vi "System State Global.vi"(7 "Notifier In":refnum<notifier>, 8 "Action":T2, 10 "State In":T1=enum."E-Stop") -> (0 "Notifier Out":refnum<notifier>, 2 "State Out":T1)   [LabVIEW 2015]
uses:
  System State Global Action.ctl
  System State.ctl
  Valve Button Mapping Global Action.ctl
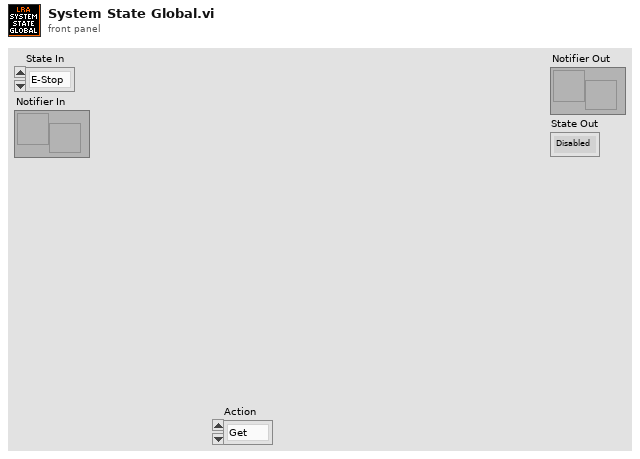
[diagram p1: front panel]
types:
  T1 = typedef "System State.ctl" = enum16{"Disabled", "E-Stop", "Standby", "Active"}
  T2 = typedef "System State Global Action.ctl" = enum16{"Get", "Set", "Initialize"}
  T3 = typedef "Valve Button Mapping Global Action.ctl" = enum16{"Get", "Set", "Init", "Reset All", "Reset to Standby"}
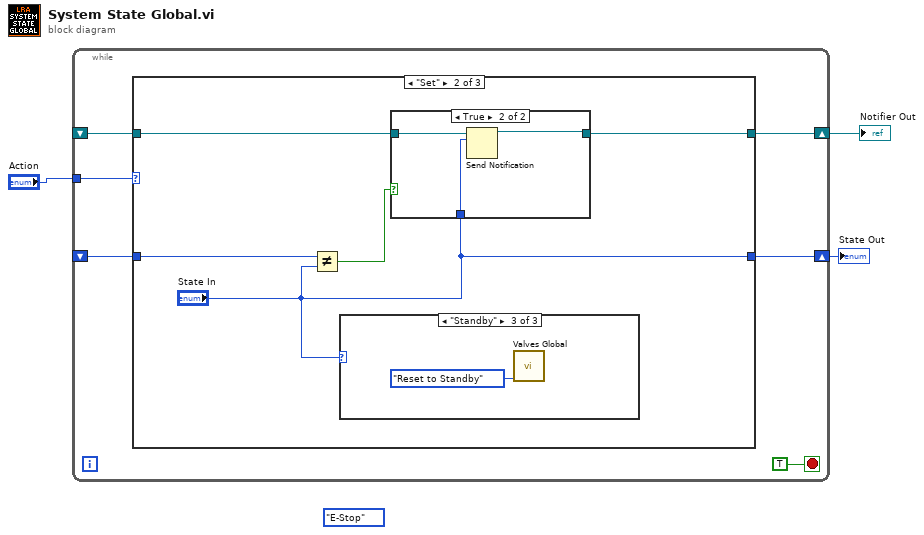
[diagram p0: block diagram]
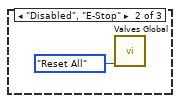
[diagram p4: hidden frame]
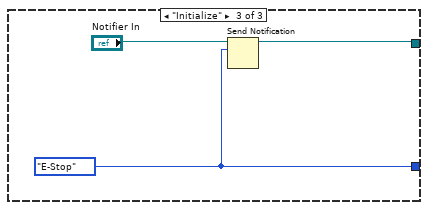
[diagram p6: hidden frame]
diagram:
  (unwired) System_State."E-Stop" ("notification")
  n1 = while {
    tunnel: "Action" -> [w8]
    shift-right: [w7] -> w1
    shift-left: _ -> [w6]
    shift-right: [w5] -> w2
    shift-left: _ -> [w4]
    stop <- TRUE stop-if-true
    n2 = case shown="\"Set\"" w8 {
      tunnel: [w11 "State In" w23] -> w7
      tunnel: w6 -> [w11 w16 _]
      tunnel: [w10 w13 w25] -> w5
      tunnel: w4 -> [w10 w14 _]
      frame "Get", Default {
      }
      frame "Set" {
        n3 = Not Equal?(x=w16, y="State In") -> (x != y?=w15:bool)
        n4 = case shown="\"Standby\"" "State In" {
          frame "Active", Default {
          }
          frame "Disabled", "E-Stop" {
            n5 = call "Valves Global.vi"("Action"=Valve_Button_Mapping_Global_Action."Reset All") -> ()  [unwired: 7 in, 4 out]
          }
          frame "Standby" {
            n6 = call "Valves Global.vi"("Action"=Valve_Button_Mapping_Global_Action."Reset to Standby") -> ()  [unwired: 7 in, 4 out]
          }
        }
        n7 = case shown="True" w15 {
          tunnel: w14 -> [w19 w22]
          tunnel: [w19 w21] -> w13
          tunnel: "State In" -> [_ w20]
          frame False {
          }
          frame True {
            n8 = Send Notification(notification=w20, notifier=w22) -> (notifier out=w21:refnum<notifier>)  [unwired: 1 in, 1 out]
          }
        }
      }
      frame "Initialize" {
        w23 = System_State."E-Stop" ("notification")
        n9 = Send Notification(notification=w23, notifier="Notifier In") -> (notifier out=w25:refnum<notifier>)  [unwired: 1 in, 1 out]
      }
    }
  }
  "Notifier Out" <- w2
  "State Out" <- w1
